vi "Save_Source_Type.vi"(8 "error in (no error)":errorcluster, 9 "index":i32, 10 "buildObject":T1, 11 "AB_Source_Exported_Assembly_VI in":refnum<class "AB_Source_Exported_Assembly_VI.lvclass">) -> (0 "error out":errorcluster, 3 "AB_Source_Exported_Assembly_VI out":refnum<class "AB_Source_Exported_Assembly_VI.lvclass">)   [LabVIEW 2020, in "AB_Source_Exported_Assembly_VI.lvclass"]
uses:
  <vilib>/AppBuilder/AB_Classes/Source/ExportedAssemblyVI/AB_Source_Exported_Assembly_VI.lvclass
  <resource>/Framework/Providers/API/ItemRef.ctl
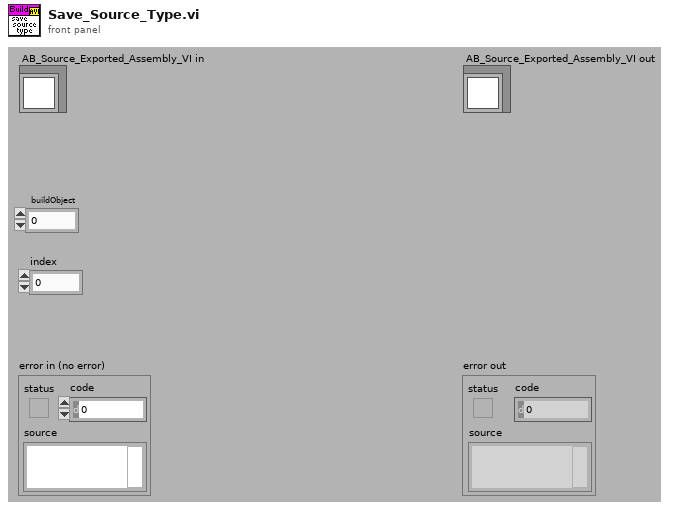
[diagram p1: front panel]
types:
  T1 = typedef "ItemRef.ctl" = u64
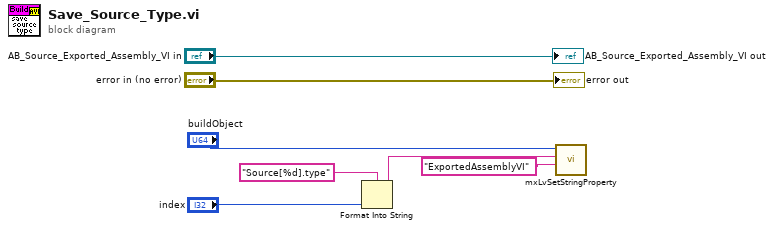
[diagram p0: block diagram]
diagram:
  n1 = Format Into String(format string="Source[%d].type", "index") -> (resulting string=w6:string)  [unwired: 2 in, 1 out]
  n2 = call <resource>:"mxLvSetStringProperty.vi"("Value (\"\")"="ExportedAssemblyVI" ("Value (\"\")"), "Tag"=w6, "Item"="buildObject") -> ()  [unwired: 2 in, 7 out]
  "error out" <- "error in (no error)"
  "AB_Source_Exported_Assembly_VI out" <- "AB_Source_Exported_Assembly_VI in"
